vi "AssertsSubpanelExecStateNotBad.vi"(11 "error in":errorcluster) -> (15 "error out":errorcluster)   [LabVIEW 2016, in "DronaTest.lvlib"]
uses:
  DronaTest.lvlib
  APIs/Stimulus/ControlValue/ValueSignalByPathString.vi
  APIs/Assert/AssertSubpanel/AssertSubpanelVIExecNotBad.vi
  <vilib>/addons/_JKI Toolkits/Caraya/classes/Test/Test.lvclass
  Drona.lvlib
  APIs/Stimulus/ControlValue/ControlValue.lvlib
  APIs/Assert/AssertSubpanel/AssertSubpanel.lvlib
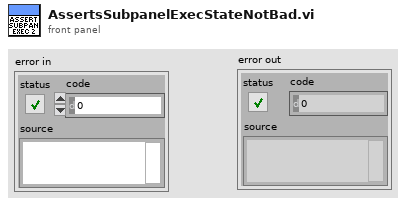
[diagram p1: front panel]
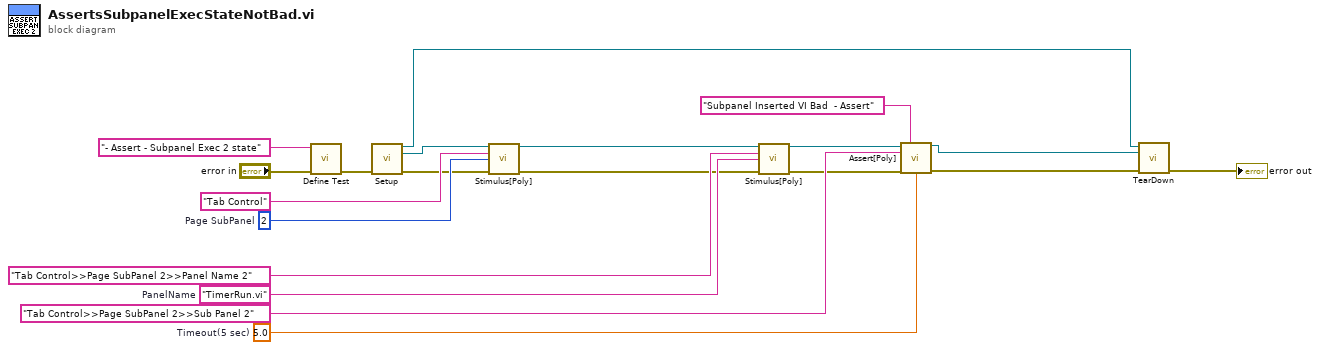
[diagram p0: block diagram]
diagram:
  w9 = 2  # Page SubPanel
  w14 = "TimerRun.vi"  # PanelName
  w16 = 5.0  # Timeout(5 sec)
  n1 = call <vilib>:"Define Test.vi"("error in (no error)"="error in", "Label (VI Title)"="- Assert - Subpanel Exec 2 state" ("string")) -> ("error out"=w11:errorcluster)  [unwired: 9 in]
  n2 = call "Setup.vi"("error in (no error)"=w11) -> ("Application Ref"=w3:refnum<vi>, "VI out"=w2:refnum<vi>, "error out"=w6:errorcluster)  [unwired: 12 in]
  n3 = call-poly "Stimulus[Poly].vi"("VI Reference In"=w2, "Control Path"="Tab Control", "Value (Signaling)"=w9, "error in"=w6) -> ("VI Reference Out"=w12:refnum<vi>, "error out"=w8:errorcluster)  [unwired: 10 in]
  n4 = call-poly "Stimulus[Poly].vi"("VI Reference In"=w12, "Control Path"="Tab Control>>Page SubPanel 2>>Panel Name 2", "Value (Signaling)"=w14, "error in"=w8) -> ("VI Reference Out"=w7:refnum<vi>, "error out"=w13:errorcluster)  [unwired: 10 in]
  n5 = call-poly "Assert[Poly].vi"("VI Reference In"=w7, "Test Label"="Subpanel Inserted VI Bad  - Assert" ("Label"), "Control Path"="Tab Control>>Page SubPanel 2>>Sub Panel 2", "Error In"=w13, "Timeout(5 sec)"=w16) -> ("VI Reference Out"=w4:refnum<vi>, "Error Out"=w15:errorcluster)  [unwired: 9 in]
  n6 = call "TearDown.vi"("Application Ref"=w3, "VI in"=w4, "error in (no error)"=w15) -> ("error out"=→"error out":errorcluster)  [unwired: 12 in]
